vi "Set Language.vi"(8 "error in":errorcluster, 10 "Target Language (current lang)":string) -> (0 "error out":errorcluster, 1 "Current Language":string)   [LabVIEW 2017, in "JKI Simple Localization.lvlib"]
doc: "Translates all VIs in registry list to the current language.\n\nTarget Language (current lang): Set this to update the current language and translate all VIs to this language. Do not wire to use the current language (If not set previously, thisi s by default the OS primary language)\n\nTo add VIs to the registry use the Register VI(s) function."
uses:
  JKI Simple Localization.lvlib
  Definitions/Private/Localization FGV Action -- Enum.ctl
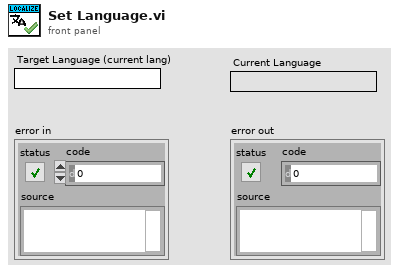
[diagram p1: front panel]
types:
  T1 = typedef "JKI Simple Localization.lvlib/Localization FGV Action -- Enum.ctl" = enum16{"Read Dictionary", "Translate VIs", "Register VI", "Get Languages", "Translate Phrase", "Translate VI", "Unregister"}
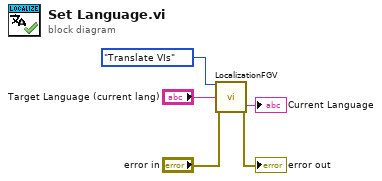
[diagram p0: block diagram]
diagram:
  n1 = call "LocalizationFGV.vi"("Action"=Localization_FGV_Action_--_Enum."Translate VIs", "Target Language"="Target Language (current lang)", "error in"="error in") -> ("Current Language"=→"Current Language":string, "error out"=→"error out":errorcluster)  [unwired: 8 in, 3 out]
